vi "Destroy CD XML Ref.vi"(8 "error in (no error)":errorcluster, 11 "Project XML Editor in":refnum<class "Project XML Editor.lvclass">) -> (0 "error out":errorcluster)   [LabVIEW 2020, in "LVLIBP CD XML Updater.lvlib" / "Project XML Editor.lvclass"]
uses:
  Project XML Editor.lvclass
  Project XML Editor.lvclass/Project XML Editor.ctl
  <vilib>/xml/Close Reference(Node).vi
  <vilib>/xml/NI_XML.lvlib
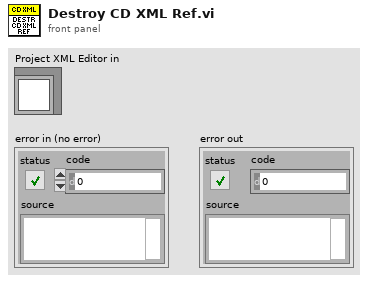
[diagram p1: front panel]
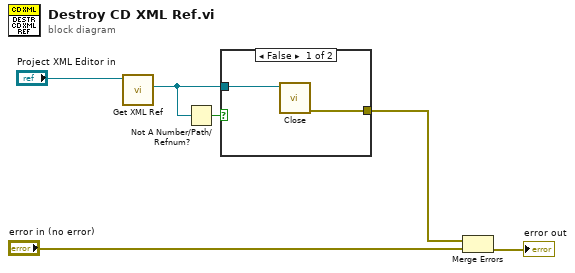
[diagram p0: block diagram]
diagram:
  n1 = call "Get XML Ref.vi"("Project XML Editor in"="Project XML Editor in") -> ("XML Ref"=w6:refnum<k20>)  [unwired: 9 in, 1 out]
  n2 = Not A Number/Path/Refnum?(number/path/refnum=w6) -> (NaN/Path/Refnum?=w5:bool)
  n3 = case shown="False" w5 {
    tunnel: [w8 _] -> w3
    tunnel: w6 -> [w7 _]
    frame False {
      n4 = call-poly <vilib>:"Close.vi"("node"=w7) -> ("error out"=w8:errorcluster)  [unwired: 8 in]
    }
    frame True {
    }
  }
  n5 = Merge Errors(w3, "error in (no error)") -> (→"error out":errorcluster)
